vi "scale_color_map.vi"(10 "Min Max":T1, 11 "Color Map In":cluster{dbl, u32}[](array[cluster])) -> (3 "Color Map Out":cluster{dbl, u32}[](array[cluster]))   [LabVIEW 2020, in "3DPC_SurfacePlot.xctl"]
uses:
  <vilib>/Native 3D Graph/xcontrol/3DPC_SurfacePlot.xctl
  <vilib>/Native 3D Graph/typedefs/range_cluster.ctl
  <vilib>/Native 3D Graph/typedefs/min_max.ctl
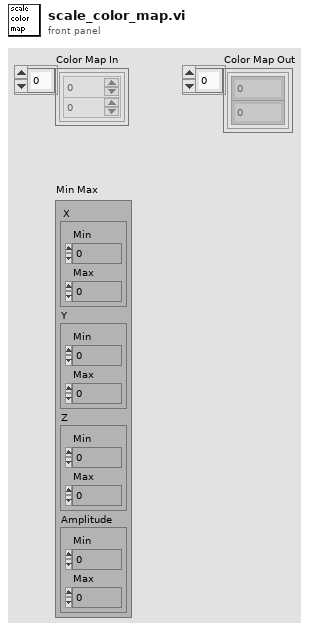
[diagram p1: front panel]
types:
  T1 = typedef "3DPC_SurfacePlot.xctl/range_cluster.ctl" = cluster{"X":T2, "Y":T2, "Z":T2, "Amplitude":T2}
  T2 = typedef "3DPC_SurfacePlot.xctl/min_max.ctl" = cluster{"Min":sgl, "Max":sgl}
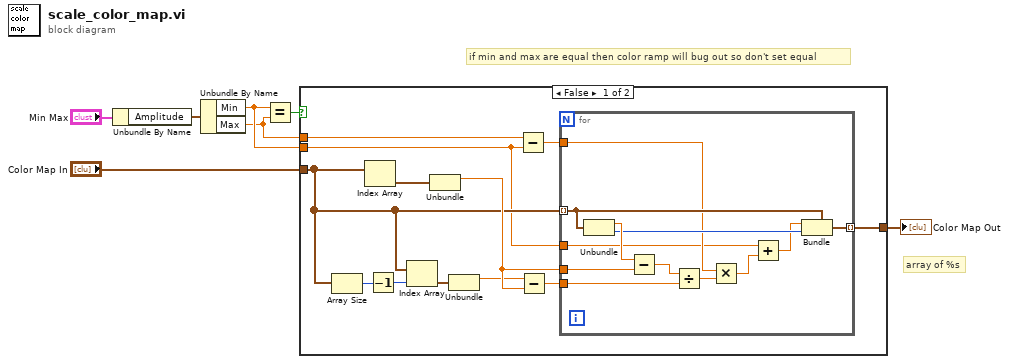
[diagram p0: block diagram]
diagram:
  # "if min and max are equal then color ramp will bug out so don't set equal"
  # "array of %s"
  n1 = Unbundle By Name("Min Max") -> ("Amplitude"=w6:T2)
  n2 = Unbundle By Name(w6) -> ("Min"=w3:sgl, "Max"=w2:sgl)
  n3 = Equal?(x=w3, y=w2) -> (x = y?=w1:bool)
  n4 = case shown="False" w1 {
    tunnel: "Color Map In" -> [w13 w32]
    tunnel: [w10 w32] -> w4
    tunnel: w3 -> [w9 _]
    tunnel: w2 -> [w8 _]
    frame False {
      n5 = Array Size(array=w13) -> (size(s)=w18:i32)
      n6 = Index Array(array=w13) -> (element=w15:cluster{dbl, u32})  [unwired: 1 in]
      n7 = Decrement(x=w18) -> (x-1=w14:i32)
      n8 = Index Array(array=w13, index=w14) -> (element=w16:cluster{dbl, u32})
      n9 = Unbundle(w15) -> (w19:dbl)  [unwired: 1 out]
      n10 = Unbundle(w16) -> (w17:dbl)  [unwired: 1 out]
      n11 = Subtract(x=w8, y=w9) -> (x-y=w11:sgl)
      n12 = Subtract(x=w17, y=w19) -> (x-y=w12:dbl)
      n13 = for {
        tunnel: w12 -> [w31]
        tunnel: w13 -> [w26] mode=indexing
        tunnel: w19 -> [w29]
        tunnel: w11 -> [w25]
        tunnel: w9 -> [w22]
        tunnel: [w20] -> w10 mode=indexing
        n14 = Unbundle(w26) -> (w30:dbl, w27:u32)
        n15 = Subtract(x=w30, y=w29) -> (x-y=w28:dbl)
        n16 = Divide(x=w28, y=w31) -> (x/y=w24:dbl)
        n17 = Multiply(x=w25, y=w24) -> (x*y=w23:dbl)
        n18 = Add(x=w22, y=w23) -> (x+y=w21:dbl)
        n19 = Bundle(cluster=w26, w21, w27) -> (w20:cluster{dbl, u32})
      }
    }
    frame True {
    }
  }
  "Color Map Out" <- w4
